vi "readCustomDeviceVersionFromXML.vi"() -> (3 "Custom device version":string)   [LabVIEW 2015, in "nipkg-utilities.lvlib"]
uses:
  nipkg-utilities.lvlib
  <vilib>/xml/Load XML File.vi
  <vilib>/xml/Close Reference(Node).vi
  <vilib>/xml/NI_XML.lvlib
  <vilib>/Wiresmith Technology/LabVIEW CLI/CLI Class/CLI.lvclass
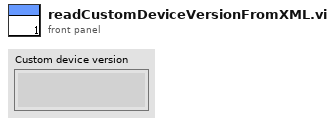
[diagram p1: front panel]
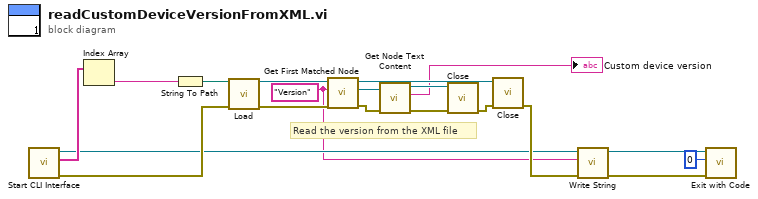
[diagram p0: block diagram]
diagram:
  w1 = "Version" ("XPath expression")
  # "Read the version from the XML file"
  n1 = call <vilib>:"Start CLI Interface.vi"() -> ("error out"=w7:errorcluster, "Custom Parameters"=w10:string[], "CLI out"=w5:refnum<class "CLI.lvclass">)  [unwired: 9 in]
  n2 = Index Array(array=w10) -> (element=w9:string)  [unwired: 1 in]
  n3 = String To Path(string=w9) -> (path=w11:path)
  n4 = call-poly <vilib>:"Load.vi"("path to XML document"=w11, "error in (no error)"=w7) -> ("DOM document out"=w17:refnum<k20>, "error out"=w16:errorcluster)  [unwired: 11 in, 1 out]
  n5 = call <vilib>:"Get First Matched Node.vi"("error in (no error)"=w16, "XPath expression"=w1, "node in"=w17) -> ("error out"=w19:errorcluster, "node result"=w18:refnum<k20>, "node out"=w13:refnum<k20>)  [unwired: 6 in]
  n6 = call <vilib>:"Get Node Text Content.vi"("error in (no error)"=w19, "node in"=w18) -> ("error out"=w14:errorcluster, "node text"=→"Custom device version":string, "node out"=w15:refnum<k20>)  [unwired: 7 in]
  n7 = call-poly <vilib>:"Close.vi"("error in (no error)"=w14, "node"=w15) -> ("error out"=w12:errorcluster)  [unwired: 7 in]
  n8 = call-poly <vilib>:"Close.vi"("error in (no error)"=w12, "node"=w13) -> ("error out"=w6:errorcluster)  [unwired: 7 in]
  n9 = call <vilib>:"Write String.vi"("error in (no error)"=w6, "Text to Write"=w1, "CLI in"=w5) -> ("error out"=w4:errorcluster, "CLI out"=w3:refnum<class "CLI.lvclass">)  [unwired: 7 in]
  n10 = call <vilib>:"Exit with Code.vi"("error in (no error)"=w4, "Exit Code (0)"=0, "CLI in"=w3) -> ()  [unwired: 8 in, 1 out]
